vi "Init-File.vi"(8 "error in (no error)":errorcluster, 11 "FileHandler in":refnum<class "RotateFileHandler.lvclass">) -> (0 "error out":errorcluster, 3 "FileHandler out":refnum<class "RotateFileHandler.lvclass">)   [LabVIEW 2024, in "RotateFileHandler.lvclass"]
uses:
  RotateFileHandler.lvclass
  RotateFileHandler.lvclass/RotateFileHandler.ctl
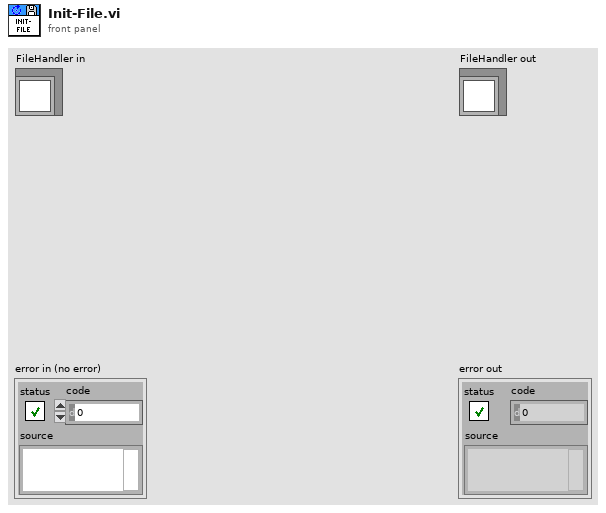
[diagram p1: front panel]
types:
  T1 = enum16{"open", "replace", "create", "open or create", "replace or create", "replace or create with confirmation"}
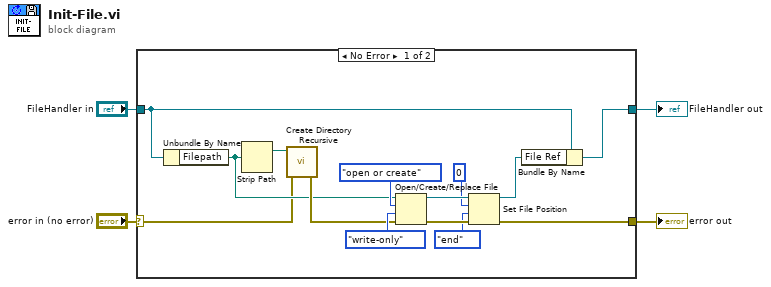
[diagram p0: block diagram]
diagram:
  n1 = case shown="No Error" "error in (no error)" {
    selector: "error in (no error)" -> [w6 w20]
    tunnel: [w5 w20] -> w3
    tunnel: [w9 w19] -> w1
    tunnel: "FileHandler in" -> [w8 w19]
    frame No Error {
      n2 = Unbundle By Name(w8) -> ("Filepath"=w10:path)
      n3 = Strip Path(path=w10) -> (stripped path=w12:path)  [unwired: 1 out]
      n4 = call <vilib>:"Create Directory Recursive.vi"("error in (no error)"=w6, "directory"=w12) -> ("error out"=w11:errorcluster)  [unwired: 3 in, 2 out]
      n5 = Open/Create/Replace File(file path (use dialog)=w10, error in=w11, operation (0:open)=T1."open or create", access (0:read/write)=enum16{"read/write", "read-only", "write-only"}."write-only") -> (refnum out=w16:refnum<file>, error out=w17:errorcluster)  [unwired: 2 in, 1 out]
      n6 = Set File Position(offset (in bytes) (0)=i64 0, refnum=w16, from (0:start)=enum16{"start", "end", "current"}."end", error in=w17) -> (refnum out=w7:refnum<file>, error out=w5:errorcluster)
      n7 = Bundle By Name(cluster=w8, "File Ref"=w7) -> (w9:refnum<class "RotateFileHandler.lvclass">)
    }
    frame Error {
    }
  }
  "error out" <- w3
  "FileHandler out" <- w1
